vi "Do Single State Callback.vi"(8 "error in (no error)":errorcluster, 9 "State":T1, 10 "State Callback":T2, 11 "Connection in":refnum<class "Connection.lvclass">) -> (0 "error out":errorcluster, 3 "Connection out":refnum<class "Connection.lvclass">)   [LabVIEW 2020, in "Stream.lvlib" / "Connection.lvclass"]
uses:
  Connection.lvclass
  Endpoint/State Callback.ctl
  Connection State.ctl
  Endpoint/Endpoint.lvclass
  Stream.lvlib
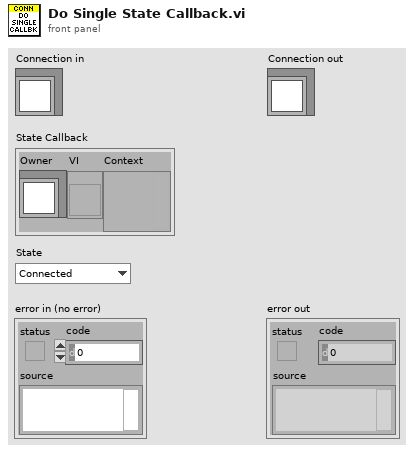
[diagram p1: front panel]
types:
  T1 = typedef "Stream.lvlib/Connection State.ctl" = enum16{"Connected", "Disconnected"}
  T2 = typedef "Stream.lvlib/Endpoint.lvclass/State Callback.ctl" = cluster{"Owner":refnum<class>, "VI":refnum<vi>, "Context":variant}
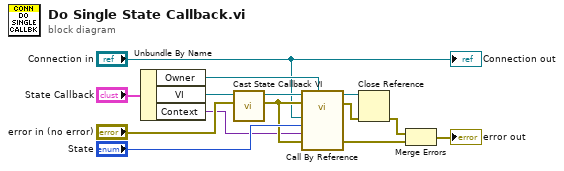
[diagram p0: block diagram]
diagram:
  n1 = Unbundle By Name("State Callback") -> ("Owner"=w9:refnum<class>, "VI"=w13:refnum<vi>, "Context"=w1:variant)
  n2 = call "Cast State Callback VI.vi"("error in (no error)"="error in (no error)", "VI Refnum"=w13) -> ("error out"=w8:errorcluster, "Casted Ref"=w11:refnum<vi>)  [unwired: 8 in]
  n3 = call-by-ref "?"(reference=w11, error in=w8, "Owner"=w9, 8:"error in (no error)"=w8, "Context"=w1, "Connection State"="State", "Connection"="Connection in") -> (reference out=w6:refnum<vi>, error out=w5:errorcluster, 0:"error out"=w7:errorcluster)  [unwired: 6 in]
  n4 = Close Reference(reference=w6, error in (no error)=w5) -> (error out=w4:errorcluster)
  n5 = Merge Errors(w4, w7) -> (→"error out":errorcluster)
  "Connection out" <- "Connection in"
